vi "SimpleREPL.vi"(11 "Microprocessor in":T1) -> ()   [LabVIEW 2016]
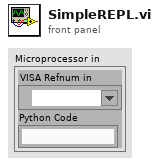
[diagram p1: front panel]
types:
  T1 = cluster{"VISA Refnum in":refnum<visa-resource-name>, "Python Code":string}
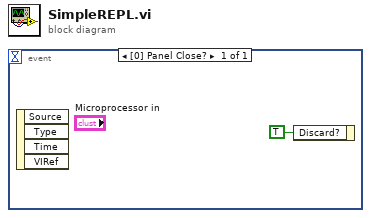
[diagram p0: block diagram]
diagram:
  n1 = event shown="[0] Panel Close?" {
    selector: _ -> [_]
    dyn-events: _ -> [_]
    timeout: _ -> [_]
    event Panel Close? {
      n2 = event-data() -> ()  [unwired: 1 in, 4 out]
      n3 = event-data("Discard?"=TRUE) -> ()  [unwired: 1 in, 1 out]
    }
  }
